vi "read result.vi"(11 "string in":string) -> (1 "Status":string, 2 "Units":string, 3 "Pressure":string)   [LabVIEW 2017]
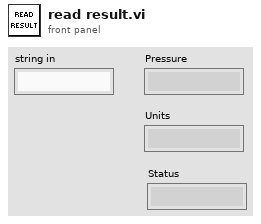
[diagram p1: front panel]
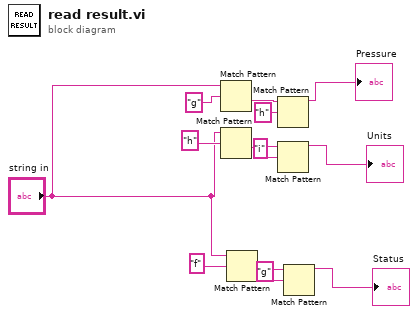
[diagram p0: block diagram]
diagram:
  n1 = Match Pattern(string="string in", regular expression="g" ("正则表达式")) -> (after substring=w9:string)  [unwired: 1 in, 3 out]
  n2 = Match Pattern(string="string in", regular expression="h" ("正则表达式")) -> (after substring=w8:string)  [unwired: 1 in, 3 out]
  n3 = Match Pattern(string="string in", regular expression="f" ("正则表达式")) -> (after substring=w4:string)  [unwired: 1 in, 3 out]
  n4 = Match Pattern(string=w9, regular expression="h" ("正则表达式")) -> (before substring=→"Pressure":string)  [unwired: 1 in, 3 out]
  n5 = Match Pattern(string=w8, regular expression="i" ("正则表达式")) -> (before substring=→"Units":string)  [unwired: 1 in, 3 out]
  n6 = Match Pattern(string=w4, regular expression="g" ("正则表达式")) -> (before substring=→"Status":string)  [unwired: 1 in, 3 out]
